vi "Tab_005_PH.vi"() -> ()   [LabVIEW 2021]
panel:
  out "Array 2":dbl[](array[numeric])
  in  "Array":dbl[](array[numeric])=[11.1, 14.2, 18.3, 22.4, 26.5]
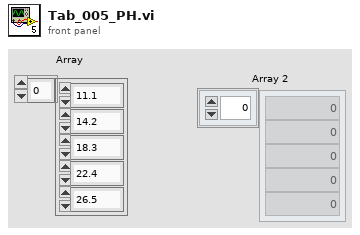
[diagram p1: front panel]
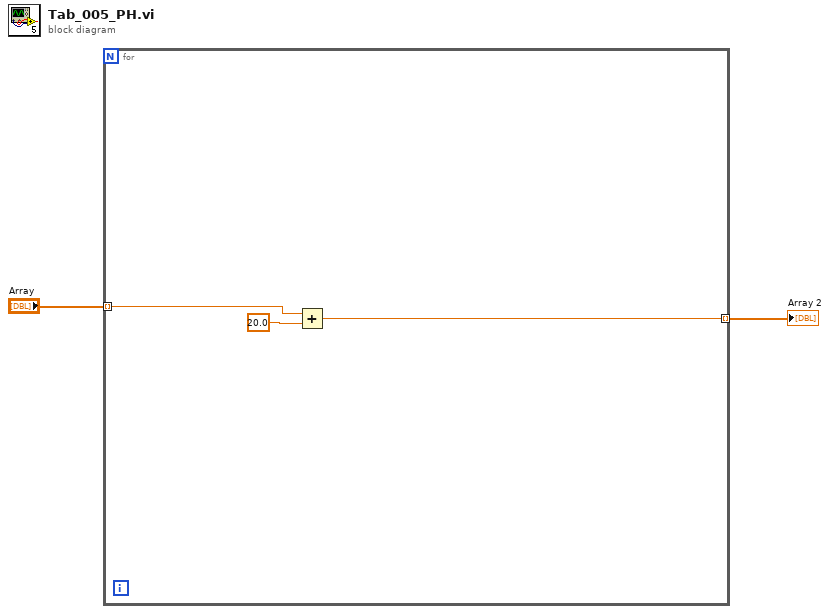
[diagram p0: block diagram]
diagram:
  n1 = for {
    tunnel: "Array" -> [w5] mode=indexing
    tunnel: [w3] -> w1 mode=indexing
    n2 = Add(x=w5, y=20.0) -> (x+y=w3:dbl)
  }
  "Array 2" <- w1
